vi "JSONfileReader.vi"(3 "error in":errorcluster, 4 "Variant":variant, 5 "ItemName":string="PickTool", 6 "FileIn":path=path "C:/Users/TTUHEP/Documents/LabVIEW/GantryPrograms/Configs/PickPlaceVacuumStates.json") -> (0 "error out":errorcluster, 1 "Data":variant, 2 "Found":bool)   [LabVIEW 2019]
uses:
  d75f7c5b-b363-447e-9fa0-018758c44a2e.vi
  <vilib>/JDP Science/JSONtext/Find Item.vi
  <vilib>/JDP Science/JSONtext/String Subset.vi
  <vilib>/JDP Science/JSONtext/Parsing/Parse Full Path or Item Name.vi
  <vilib>/JDP Science/JSONtext/Next JSON Value.vi
  <vilib>/JDP Science/JSONtext/support/Error Cluster From Code.vi
  <vilib>/JDP Science/JSONtext/Offset/Find Item Locations by Path.vi
  <vilib>/JDP Science/JSONtext/JSON text to Variant.vi
  <vilib>/JDP Science/JSONtext/LVClass Serializer/JSONtext LVClass Serializer.lvclass
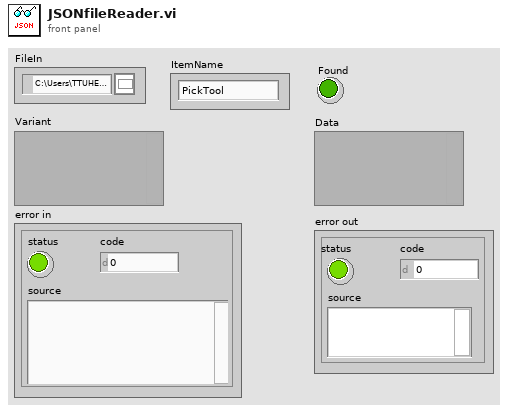
[diagram p1: front panel]
types:
  T1 = enum16{"open", "replace", "create", "open or create", "replace or create", "replace or create with confirmation"}
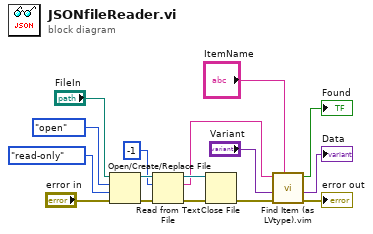
[diagram p0: block diagram]
diagram:
  n1 = Open/Create/Replace File(file path (use dialog)="FileIn", error in="error in", operation (0:open)=T1."open", access (0:read/write)=enum16{"read/write", "read-only", "write-only"}."read-only") -> (refnum out=w16:refnum<file>, error out=w15:errorcluster)  [unwired: 2 in, 1 out]
  n2 = Read from Text File(file (use dialog)=w16, count=-1, error in=w15) -> (refnum out=w13:refnum<file>, text=w6:string, error out=w12:errorcluster)  [unwired: 1 in, 1 out]
  n3 = Close File(refnum=w13, error in=w12) -> (error out=w2:errorcluster)  [unwired: 1 out]
  n4 = call "Find Item (as LVtype).vim"("$Path or Item Name"="ItemName", "error in (no error)"=w2, "Data Type and Default Value"="Variant", "JSON"=w6) -> ("error out"=→"error out":errorcluster, "Data"=→"Data":variant, "Found"=→"Found":bool)  [unwired: 4 in, 1 out]
